vi "Controller2.vi"(4 "process variable":dbl format="%.2f", 8 "setpoint":dbl format="%.2f", 9 "auto_man":bool, 10 "man_output u [V]":dbl, 11 "PID gains":T1) -> (3 "output":dbl)   [LabVIEW 2018]
uses:
  <vilib>/addons/control/pid/pid.llb/PID Advanced (DBL).vi
  <vilib>/addons/control/pid/NI_PID_pid.lvlib
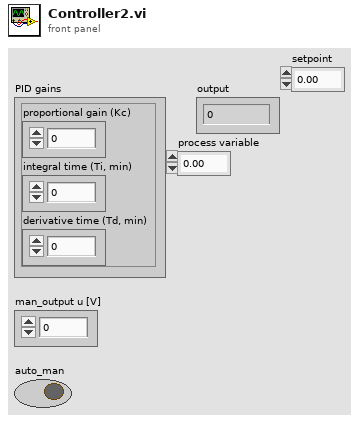
[diagram p1: front panel]
types:
  T1 = cluster{"proportional gain (Kc)":dbl, "integral time (Ti, min)":dbl, "derivative time (Td, min)":dbl}
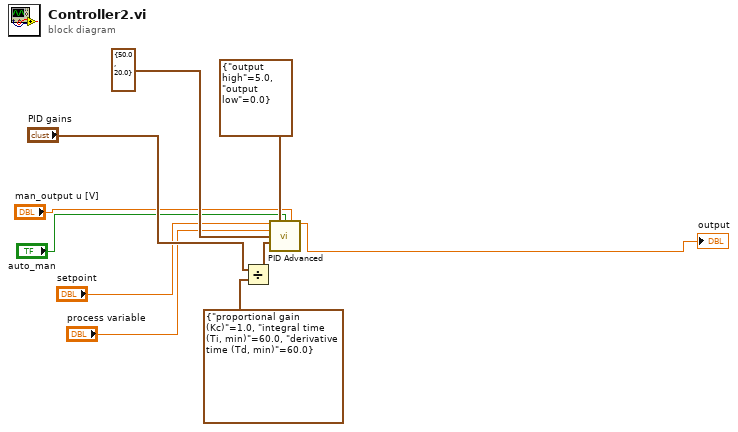
[diagram p0: block diagram]
diagram:
  n1 = Divide(x="PID gains", y=T1 {"proportional gain (Kc)"=1.0, "integral time (Ti, min)"=60.0, "derivative time (Td, min)"=60.0}) -> (x/y=w9:T1)
  n2 = call-poly <vilib>:"PID Advanced.vi"("setpoint"="setpoint", "output range"=cluster{"output high":dbl, "output low":dbl} {"output high"=5.0, "output low"=0.0}, "auto? (T)"="auto_man", "manual control"="man_output u [V]", "process variable"="process variable", "setpoint range"=cluster{"setpoint high":dbl, "setpoint low":dbl} {"setpoint high"=50.0, "setpoint low"=20.0}, "PID gains"=w9) -> ("output"=→"output":dbl)  [unwired: 7 in, 1 out]
